vi "goToabsXY.vi"(8 "error in":errorcluster, 10 "Y position":dbl, 11 "X position":dbl) -> (0 "error out":errorcluster)   [LabVIEW 2014]
doc: "André Romero - 2023\nandretec@ifsc.usp.br\nIFSC - USP"
uses:
  Global Motors.vi
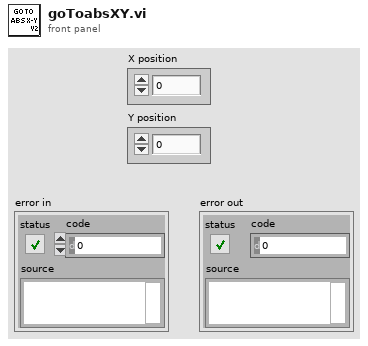
[diagram p1: front panel]
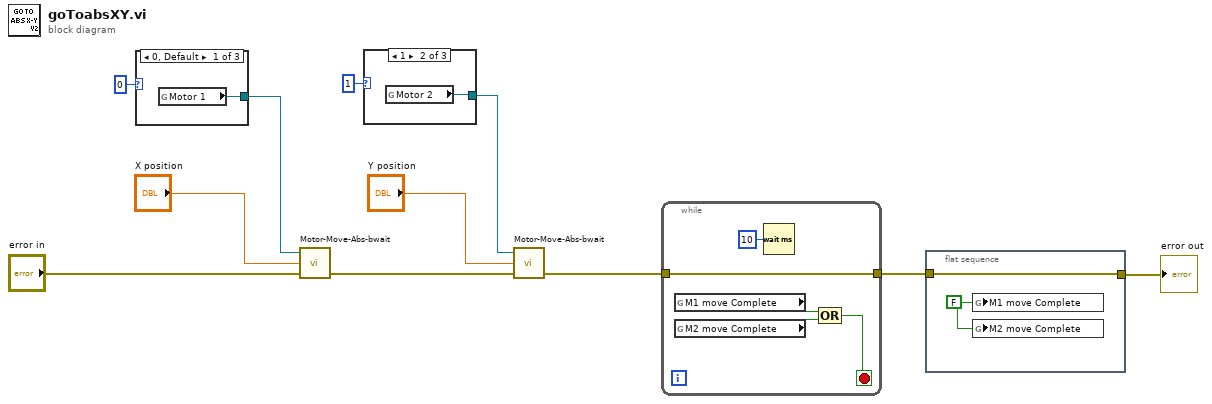
[diagram p0: block diagram]
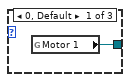
[diagram p2: hidden frame]
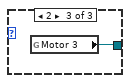
[diagram p3: hidden frame]
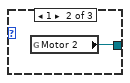
[diagram p4: hidden frame]
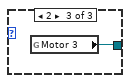
[diagram p5: hidden frame]
diagram:
  n1 = case shown="0, Default" u16 0 ("Axis") {
    tunnel: [w12 w13 w14] -> w11
    frame 0, Default {
      n2 = global read "Global Motors.vi" "Motor 1"() -> (w12:refnum<k7>)
    }
    frame 1 {
      n3 = global read "Global Motors.vi" "Motor 2"() -> (w13:refnum<k7>)
    }
    frame 2 {
      n4 = global read "Global Motors.vi" "Motor 3"() -> (w14:refnum<k7>)
    }
  }
  n5 = call "Motor-Move-Abs-bwait.vi"("error"="error in", "Posição"="X position", "MG17Motor A"=w11) -> ("error out"=w6:errorcluster)  [unwired: 1 in, 1 out]
  n6 = case shown="1" u16 1 ("Axis") {
    tunnel: [w15 w16 w17] -> w1
    frame 0, Default {
      n7 = global read "Global Motors.vi" "Motor 1"() -> (w15:refnum<k7>)
    }
    frame 1 {
      n8 = global read "Global Motors.vi" "Motor 2"() -> (w16:refnum<k7>)
    }
    frame 2 {
      n9 = global read "Global Motors.vi" "Motor 3"() -> (w17:refnum<k7>)
    }
  }
  n10 = call "Motor-Move-Abs-bwait.vi"("error"=w6, "Posição"="Y position", "MG17Motor A"=w1) -> ("error out"=w3:errorcluster)  [unwired: 1 in, 1 out]
  n11 = while {
    tunnel: w3 -> [w22]
    tunnel: [w22] -> w2
    stop <- w19 stop-if-true
    n12 = global read "Global Motors.vi" "M1 move Complete"() -> (w21:bool)
    n13 = global read "Global Motors.vi" "M2 move Complete"() -> (w20:bool)
    n14 = Wait (ms)(milliseconds to wait=u32 10) -> ()  [unwired: 1 out]
    n15 = Compound Arithmetic op=OR(w21, w20) -> (w19:bool)
  }
  n16 = flat-sequence {
    tunnel: w2 -> [w24]
    tunnel: [w24] -> w10
    frame #0 {
      w23 = FALSE ("M1 move Complete")
      n17 = global write "Global Motors.vi" "M1 move Complete"(w23) -> ()
      n18 = global write "Global Motors.vi" "M2 move Complete"(w23) -> ()
    }
  }
  "error out" <- w10
